vi "Calc XYZ_kj.vi"(8 "theta_j":dbl, 9 "j":i32, 10 "XYZbar_k":dbl[](array[numeric]), 11 "Analytical Serial Arm Class in":refnum<class "NI_Robotics_Analytical Serial Arm Class.lvclass">) -> (1 "Xstar_ij":dbl, 2 "XYZ_ij":dbl[](array[numeric]), 3 "Analytical Serial Arm Class out":refnum<class "NI_Robotics_Analytical Serial Arm Class.lvclass">)   [LabVIEW 2017, in "NI_Robotics_Analytical Serial Arm Class.lvclass"]
uses:
  <vilib>/robotics/Kinematics/Analytical/Generic/NI_Robotics_Analytical Serial Arm Class.lvclass
  c:/Program Files (x86)/National Instruments/LabVIEW 2017/vi.lib/robotics/Kinematics/Robot/NI_Robotics_Serial Robot Arm.lvclass
  <vilib>/robotics/Kinematics/Link/NI_Robotics_Link.lvclass/NI_Robotics_Link.ctl
  <vilib>/robotics/Kinematics/Link/Get Kinematic Parameters.vi
  <vilib>/robotics/Kinematics/Analytical/Generic/Accessors/Read alpha_n0.vi
  <vilib>/robotics/Kinematics/Robot/Get Links.vi
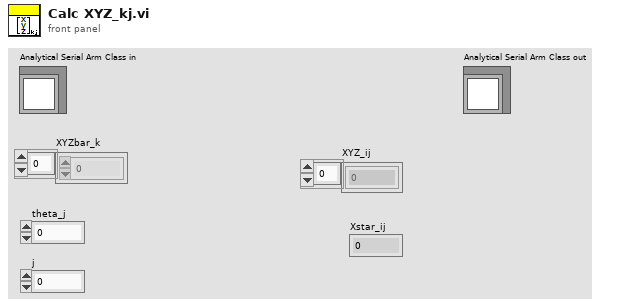
[diagram p1: front panel]
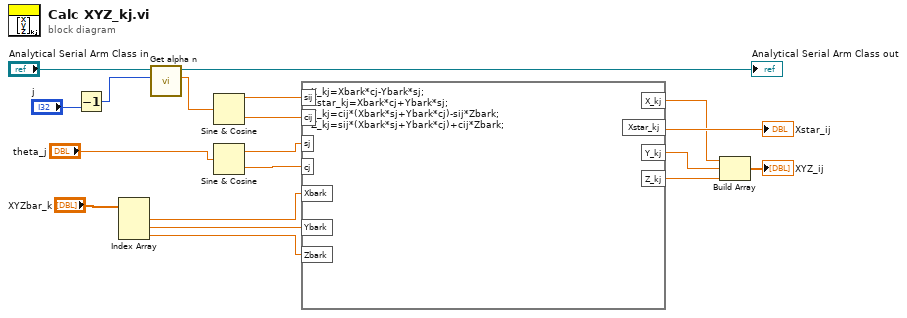
[diagram p0: block diagram]
diagram:
  n1 = Decrement(x="j") -> (x-1=w1:i32)
  n2 = Index Array(array="XYZbar_k") -> (element #1=w4:dbl, element #2=w3:dbl, element #3=w2:dbl)  [unwired: 3 in]
  n3 = call <vilib>:"Get alpha n.vi"("n"=w1, "Analytical Serial Arm Class in"="Analytical Serial Arm Class in") -> ("alpha n"=w16:dbl, "Analytical Serial Arm Class out"=→"Analytical Serial Arm Class out":refnum<class "NI_Robotics_Analytical Serial Arm Class.lvclass">)  [unwired: 8 in]
  n4 = Sine & Cosine(0:w16) -> (1:w13:dbl, 2:w12:dbl)
  n5 = Sine & Cosine(0:"theta_j") -> (1:w11:dbl, 2:w10:dbl)
  n6 = formula code="X_kj=Xbark*cj-Ybark*sj;\nXstar_kj=Xbark*cj+Ybark*sj;\nY_kj=cij*(Xbark*sj+Ybark*cj)-sij*Zbark;\nZ_kj=sij*(Xbark*sj+Ybark*cj)+cij*Zbark;"("sij"=w13, "cij"=w12, "sj"=w11, "cj"=w10, "Xbark"=w4, "Ybark"=w3, "Zbark"=w2) -> ("X_kj"=w7:dbl, "Xstar_kj"=→"Xstar_ij":dbl, "Y_kj"=w8:dbl, "Z_kj"=w9:dbl)
  n7 = Build Array(w7, w8, w9) -> (→"XYZ_ij":dbl[])
